vi "Polling Core.vi"(8 "Error In":errorcluster, 11 "CS++DMM in":refnum<class "CS++DMM.lvclass">) -> (0 "Error Out":errorcluster, 3 "CS++DMM out":refnum<class "CS++DMM.lvclass">)   [LabVIEW 2015, in "CS++DMM.lvlib" / "CS++DMM.lvclass"]
doc: "Implement the pseudo-periodic action in your override.vi."
uses:
  CS++DMM.lvclass
  CS++DMM.lvclass/CS++DMM.ctl
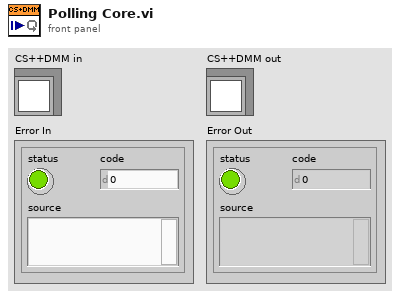
[diagram p1: front panel]
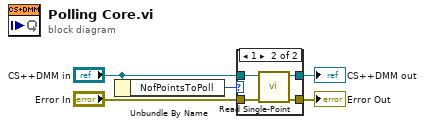
[diagram p0: block diagram]
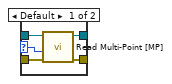
[diagram p2: hidden frame]
diagram:
  n1 = Unbundle By Name("CS++DMM in") -> ("NofPointsToPoll"=w3:i32)
  n2 = case shown="1" w3 {
    selector: w3 -> [w6 _]
    tunnel: "Error In" -> [w9 w13]
    tunnel: "CS++DMM in" -> [w10 w14]
    tunnel: [w7 w12] -> w2
    tunnel: [w8 w11] -> w1
    frame Default {
      n3 = call "Read Multi-Point [MP].vi"("error in (no error)"=w9, "array size"=w6, "CS++DMM in"=w10) -> ("error out"=w8:errorcluster, "CS++DMM out"=w7:refnum<class "CS++DMM.lvclass">)  [unwired: 5 in, 2 out]
    }
    frame 1 {
      n4 = call "Read Single-Point.vi"("error in (no error)"=w13, "CS++DMM in"=w14) -> ("error out"=w11:errorcluster, "CS++DMM out"=w12:refnum<class "CS++DMM.lvclass">)  [unwired: 7 in, 1 out]
    }
  }
  "Error Out" <- w1
  "CS++DMM out" <- w2
